vi "oa_Compute DC Gap Value (1 Channel).vi"(0 "signal in":dbl[](array[numeric]), 1 "reset?":bool=TRUE, 2 "select reference data":T1(ring), 5 "dt":dbl, 7 "start points":i32[](array[numeric]), 9 "durations":i32[](array[numeric]), 11 "error in":errorcluster, 12 "averaging type":enum16{"Linear", "Exponential"}(ring), 13 "window":T2(ring)) -> (4 "DC value":dbl, 15 "error out":errorcluster)   [LabVIEW 2017, in "SoundVib_RefDataProcess.lvlib"]
uses:
  <vilib>/addons/Sound and Vibration/Order Analysis/Referece Data Processing/SoundVib_RefDataProcess.lvlib
  <vilib>/measure/madcrms.llb/Basic Averaged DC-RMS for 1 Chan.vi
  <vilib>/measure/NI_MAPro.lvlib
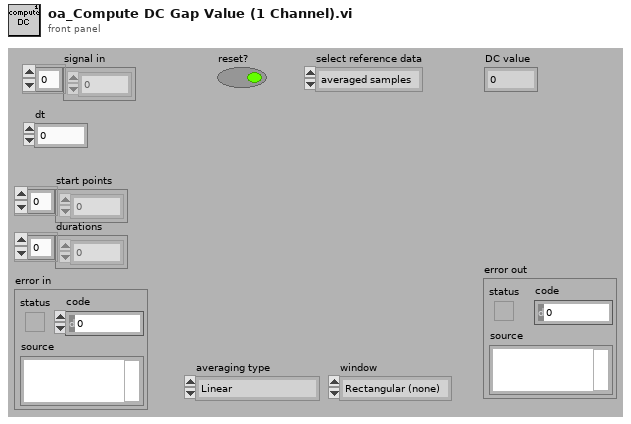
[diagram p1: front panel]
types:
  T1 = enum16{"averaged samples", "initial samples", "final samples"}
  T2 = enum16{"Rectangular (none)", "Hanning", "Low side lobe"}
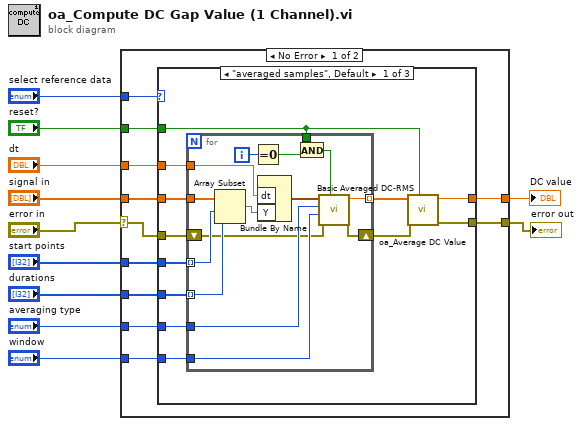
[diagram p0: block diagram]
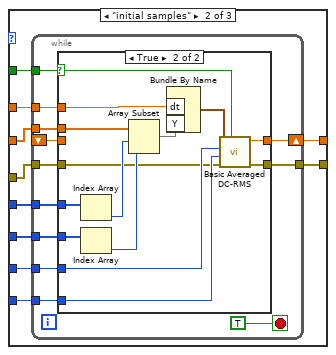
[diagram p2: hidden frame]
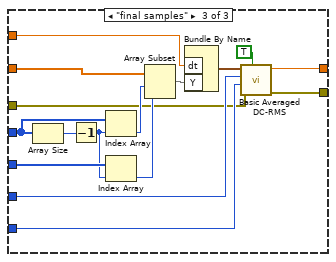
[diagram p4: hidden frame]
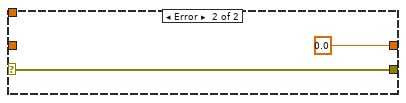
[diagram p5: hidden frame]
diagram:
  n1 = case shown="No Error" "error in" {
    selector: "error in" -> [w14 w105]
    tunnel: "start points" -> [w13 _]
    tunnel: [w22 w105] -> w10
    tunnel: [w21 0.0 ("DC value")] -> w9
    tunnel: "window" -> [w20 _]
    tunnel: "averaging type" -> [w19 _]
    tunnel: "reset?" -> [w18 _]
    tunnel: "signal in" -> [w17 _]
    tunnel: "durations" -> [w16 _]
    tunnel: "select reference data" -> [w15 _]
    tunnel: "dt" -> [w12 _]
    frame No Error {
      n2 = case shown="\"averaged samples\", Default" w15 {
        tunnel: w13 -> [w34 w55 w98]
        tunnel: w16 -> [w33 w54 w96]
        tunnel: w17 -> [w32 w56 w94]
        tunnel: w18 -> [w25 w59 _]
        tunnel: w19 -> [w24 w58 w102]
        tunnel: w20 -> [w30 w57 w101]
        tunnel: w14 -> [w31 w53 w91]
        tunnel: [w26 w52 w99] -> w21
        tunnel: [w27 w51 w100] -> w22
        tunnel: w12 -> [w23 w50 w88]
        frame "averaged samples", Default {
          n3 = for {
            tunnel: w34 -> [w40] mode=indexing
            tunnel: w33 -> [w39] mode=indexing
            tunnel: w32 -> [w41]
            shift-right: [w49] -> w28
            shift-left: w31 -> [w38]
            tunnel: w25 -> [w44]
            tunnel: w24 -> [w48]
            tunnel: w30 -> [w47]
            tunnel: [w42] -> w29 mode=indexing
            tunnel: w23 -> [w36]
            i -> [w46]
            n4 = Array Subset(array=w41, index=w40, length=w39) -> (w37:dbl[])
            n5 = Equal To 0?(x=w46) -> (x = 0?=w45:bool)
            n6 = Bundle By Name("dt"=w36, "Y"=w37) -> (w35:waveform(dbl))  [unwired: 1 in]
            n7 = And(x=w44, y=w45) -> (x .and. y?=w43:bool)
            n8 = call-poly <vilib>:"Basic Averaged DC-RMS.vi"("reset"=w43, "error in (no error)"=w38, "window"=w47, "averaging type"=w48, "signal in"=w35) -> ("error out"=w49:errorcluster, "DC value"=w42:dbl)  [unwired: 3 in, 2 out]
          }
          n9 = call <vilib>:"oa_Average DC Value.vi"("reset?"=w25, "error in"=w28, "value in"=w29) -> ("error out"=w27:errorcluster, "value"=w26:dbl)  [unwired: 7 in]
        }
        frame "initial samples" {
          n10 = while {
            tunnel: w59 -> [w64]
            tunnel: w58 -> [w71]
            tunnel: w57 -> [w70]
            tunnel: w56 -> [w69]
            tunnel: w55 -> [w68]
            tunnel: w54 -> [w67]
            tunnel: w53 -> [w66]
            shift-right: [w63] -> w52
            shift-left: _ -> [w62]
            tunnel: [w61] -> w51
            tunnel: w50 -> [w60]
            stop <- TRUE stop-if-true
            n11 = case shown="True" w64 {
              selector: w64 -> [_ w84]
              tunnel: w71 -> [_ w87]
              tunnel: w70 -> [_ w86]
              tunnel: w69 -> [_ w80]
              tunnel: w68 -> [_ w85]
              tunnel: w67 -> [_ w81]
              tunnel: w66 -> [w72 w77]
              tunnel: [w73 w83] -> w63
              tunnel: w62 -> [w73 _]
              tunnel: [w72 w82] -> w61
              tunnel: w60 -> [_ w75]
              frame False {
              }
              frame True {
                n12 = Index Array(array=w85) -> (element=w79:i32)  [unwired: 1 in]
                n13 = Index Array(array=w81) -> (element=w78:i32)  [unwired: 1 in]
                n14 = Array Subset(array=w80, index=w79, length=w78) -> (w76:dbl[])
                n15 = Bundle By Name("dt"=w75, "Y"=w76) -> (w74:waveform(dbl))  [unwired: 1 in]
                n16 = call-poly <vilib>:"Basic Averaged DC-RMS.vi"("reset"=w84, "error in (no error)"=w77, "window"=w86, "averaging type"=w87, "signal in"=w74) -> ("error out"=w82:errorcluster, "DC value"=w83:dbl)  [unwired: 3 in, 2 out]
              }
            }
          }
        }
        frame "final samples" {
          n17 = Array Size(array=w98) -> (size(s)=w97:i32)
          n18 = Decrement(x=w97) -> (x-1=w95:i32)
          n19 = Index Array(array=w98, index=w95) -> (element=w93:i32)
          n20 = Index Array(array=w96, index=w95) -> (element=w92:i32)
          n21 = Array Subset(array=w94, index=w93, length=w92) -> (w90:dbl[])
          n22 = Bundle By Name("dt"=w88, "Y"=w90) -> (w89:waveform(dbl))  [unwired: 1 in]
          n23 = call-poly <vilib>:"Basic Averaged DC-RMS.vi"("reset"=TRUE, "error in (no error)"=w91, "window"=w101, "averaging type"=w102, "signal in"=w89) -> ("error out"=w100:errorcluster, "DC value"=w99:dbl)  [unwired: 3 in, 2 out]
        }
      }
    }
    frame Error {
    }
  }
  "error out" <- w10
  "DC value" <- w9
